vi "Neutral_ScanAgilentTrim_20170616.vi"(0 "Agilent E3631A Settings":T6={"VISA resource name"="GPIB0::5::INSTR", "Voltage Set (6V max)"=6.0, "Current Set (5A max)"=0.007, "Voltage Set (25V max)"=25.0, "Current Set (1A max)"=0.225, "Voltage Set (-25V max)"=25.0, "Current Set (1A max)"=0.225, "6V Switch"=FALSE, "+25V Switch"=FALSE, "-25V Switch"=FALSE, "Agilent E3631A Measurements"={"6V Actual Voltage Level (V)"=0.03231557, "6V Actual Current Level (A)"=0.01701259, "25V Actual Voltage Level (V)"=0.4256878, "25V Actual Current Level (A)"=0.2772881, "-25V Actual Current Level (A)"=0.0, "-25V Actual Voltage Level (V)"=0.0}, "Triggered Agilent Settings"={"Trigger \nDelay (s)"=3.0, "Enable +6V Channel"=TRUE, "+6V Current"=0.02, "Enable -25V Channel"=FALSE, "-25V Current"=0.0, "Enable +25V Channel"=TRUE, "+25V Current"=0.275}, "Auto Program Agilent"=FALSE, "Agilent Software Trigger"=FALSE} {"Triggered Agilent Settings"."Trigger \nDelay (s)" min=0.0 max=3600.0 step=1.0 format="%.2f"; "Agilent E3631A Measurements"."-25V Actual Current Level (A)" format="%.3g"; "Agilent E3631A Measurements"."-25V Actual Voltage Level (V)" format="%.3g"; "Agilent E3631A Measurements"."25V Actual Current Level (A)" format="%.3g"; "Agilent E3631A Measurements"."25V Actual Voltage Level (V)" format="%.3g"; "Agilent E3631A Measurements"."6V Actual Current Level (A)" format="%.3g"; "Agilent E3631A Measurements"."6V Actual Voltage Level (V)" format="%.3g"; "Current Set (1A max)" format="%.3g"; "Voltage Set (-25V max)" format="%.3g"; "Current Set (1A max)" format="%.3g"; "Voltage Set (25V max)" format="%.3g"; "Current Set (5A max)" format="%.3g"; "Voltage Set (6V max)" format="%.3g"}, 1 "Scan Parameters":T1={"Initial Values"=[81.5, 1.0, -0.1, 1.0], "Final Values"=[82.5, 3.0, 0.075, 5.0], "Step Sizes"=[0.015, 1.0, 0.025, 1.0], "Parameters to Change"=[enum."Synth Frequency", enum."Dummy Variable", enum."Red Mot 87 Initial Voltage", enum."Dummy Variable"], "Channels to Change"=[2, 0, 7, 0], "Number of Parameters to Scan"=2, "Parameter Nickname (no spaces)"=["", "ScanNo-", "Z-", "ScanNo-"], "Scan Base Name"="88Sr_3P1Spec_BFieldZero_X-0.02A_Y-0.277A_Z-0.6A_", "Raw_Data Folder"=path "\\\\mercury\\Neutral_Experiment/Raw_Data/2017.06.15", "ROI Parameters"={"Background Radius"=150.0, "Atom Radius"=120.0, "X Center"=365.0, "Y Center"=460.0}, "Drop Time (ms)"=17.0, "Phases To Change"=[1, 0, 2, 0], "Scan Pulseblaster Channel With Parameter"={"Change PB Time Toggle"=FALSE, "PB Channel"=10.0, "Parameter Number"=0.0}, "Preserve Waveform\nContinuity"=FALSE, "Generated Array Type"=enum."Default (old way)", "Master Batch Third Column"=0.277, "Master Batch Fourth Column"=0.0, "Master Batch Fifth Column"=0.0, "Current Param. Values"=[81.5, 1.0]} {"Current Param. Values" format="%^#.3e"; "Drop Time (ms)" min=1.0; "Number of Parameters to Scan" min=1}, 2 "Control Reference Cluster Input":T5, 3 "error in (no error)":errorcluster={"status"=FALSE, "code"=0, "source"="gettemp.vi: No error - function call successful"}) -> (10 "Error Out":errorcluster)   [LabVIEW 2016]
uses:
  Controls/Agilent E3631A/Settings_Control.ctl
  Controls/Agilent E3631A/Measurement_Indicator.ctl
  Controls/Agilent E3631A/Trigger_Settings.ctl
  Controls/ScanParameters/ScanParametersPanel.ctl
  Controls/ScanParameters/ParameterToChange.ctl
  Controls/ScanParameters/ROI_set.ctl
  Controls/ScanParameters/ScanPBandParam.ctl
panel:
  # "Select a PB Channel to set with a phase time for evaporation or whatever"
  # "Since the Agilent is slow to communicate the program will skip programming if the \"Auto Program Agilent\" switch is disabled.  If \"Auto Program\" is enabled the settings to the far left are used to program the Agilent.\n\nAdditionally, the Agilent has an internal software trigger that can a single channel between two current setpoints. The clock is not referenced to the Pulseblaster so be careful with timing when using the Triggered Agilent Settings. To enabled this mode use the \"Agilent Software Trigger\" swithc.\n\nUse the \"Program Agilent\" button to perform a one-time write (with settings on the far left) to avoid having the slow response of the supply during data scans.\n\nNOTE: When setting only current values the program will default to setting the maximum allowed voltage for a given channel."
  # "6V (2017.06.15)\n\nReported Current = \nSet Cur - 0.003A\n\nActual Current = \nSet Cur - 0.0015A"
  # "+25V (2017.06.15)\n\nReported Current = \nSet Cur + 0.002A\n\nActual Current = \nSet Cur + 0.002A"
  # "-25V (2017.06.15)\n\nReported Current = \nSet Cur\n\nActual Current = \nSet Cur"
  # "Beware of the offset in set, reported and actual current from Agilent channels. Below are corrections measured for each channel"
  # "--25V  Measurements"
  # "+25V  Measurements"
  # "6V  Measurements"
  # "-25V Output Settings"
  # "+25V Output Settings"
  # "6V Output Settings"
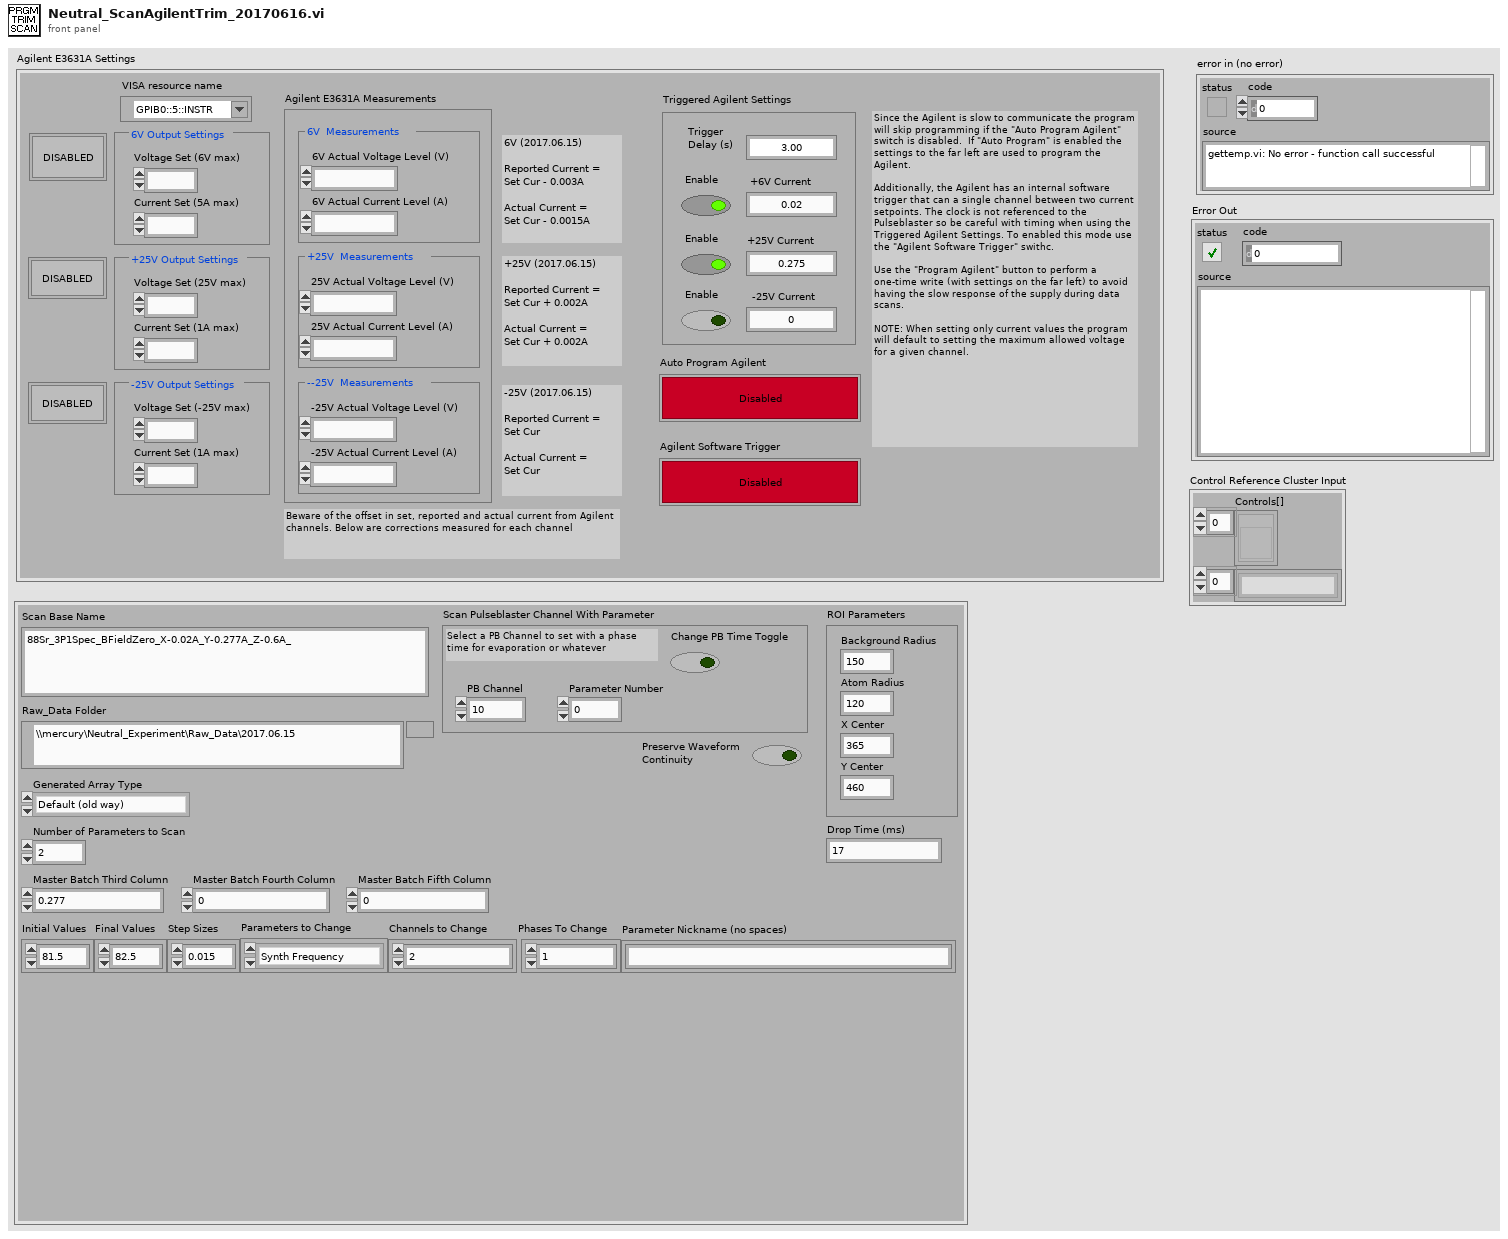
[diagram p1: front panel]
types:
  T1 = typedef "ScanParametersPanel.ctl" = cluster{"Initial Values":dbl[], "Final Values":dbl[], "Step Sizes":dbl[], "Parameters to Change":T2[], "Channels to Change":u32[], "Number of Parameters to Scan":i32, "Parameter Nickname (no spaces)":string[], "Scan Base Name":string, "Raw_Data Folder":path, "ROI Parameters":T3, "Drop Time (ms)":dbl, "Phases To Change":u32[], "Scan Pulseblaster Channel With Parameter":T4, "Preserve Waveform\nContinuity":bool, "Generated Array Type":enum16{"Custom Array From File", "Default (old way)"}, "Master Batch Third Column":dbl, "Master Batch Fourth Column":dbl, "Master Batch Fifth Column":dbl, "Current Param. Values":dbl[]}
  T2 = typedef "ParameterToChange.ctl" = enum16{"Dummy Variable", "Synth Amplitude", "Synth Frequency", "Synth Phase", "ODT Params Phase Time", "ODT Params Tau", "ODT Params Final Voltage", "ODT Params Initial Voltage", "ODT Params Eta", "Red Mot 88 Phase Time", "Red Mot 87 Phase Time", "Red Mot 88 Final Voltage", "Red Mot 88 Initial Voltage", "Red Mot 87 Final Voltage", "Red Mot 87 Initial Voltage", "PulseBlaster", "6713 Voltage", "Green Lattice Phase Time", "Green Lattice Initial Voltage", "Green Lattice Final Voltage", "Agilent Current Setpoint", "FPGA - Constant Op - Set", "FPGA - Bool Op - Output HI", "FPGA - Bool Op - Output LO", "FPGA - Custom Op"}
  T3 = typedef "ROI_set.ctl" = cluster{"Background Radius":dbl, "Atom Radius":dbl, "X Center":dbl, "Y Center":dbl}
  T4 = typedef "ScanPBandParam.ctl" = cluster{"Change PB Time Toggle":bool, "PB Channel":dbl, "Parameter Number":dbl}
  T5 = cluster{"Controls[]":refnum<vi>[], "Control Names":string[]}
  T6 = typedef "Settings_Control.ctl" = cluster{"VISA resource name":refnum<visa-resource-name>, "Voltage Set (6V max)":dbl, "Current Set (5A max)":dbl, "Voltage Set (25V max)":dbl, "Current Set (1A max)":dbl, "Voltage Set (-25V max)":dbl, "Current Set (1A max)":dbl, "6V Switch":bool, "+25V Switch":bool, "-25V Switch":bool, "Agilent E3631A Measurements":T7, "Triggered Agilent Settings":T8, "Auto Program Agilent":bool, "Agilent Software Trigger":bool}
  T7 = typedef "Measurement_Indicator.ctl" = cluster{"6V Actual Voltage Level (V)":dbl, "6V Actual Current Level (A)":dbl, "25V Actual Voltage Level (V)":dbl, "25V Actual Current Level (A)":dbl, "-25V Actual Current Level (A)":dbl, "-25V Actual Voltage Level (V)":dbl}
  T8 = typedef "Trigger_Settings.ctl" = cluster{"Trigger \nDelay (s)":dbl, "Enable +6V Channel":bool, "+6V Current":dbl, "Enable -25V Channel":bool, "-25V Current":dbl, "Enable +25V Channel":bool, "+25V Current":dbl}
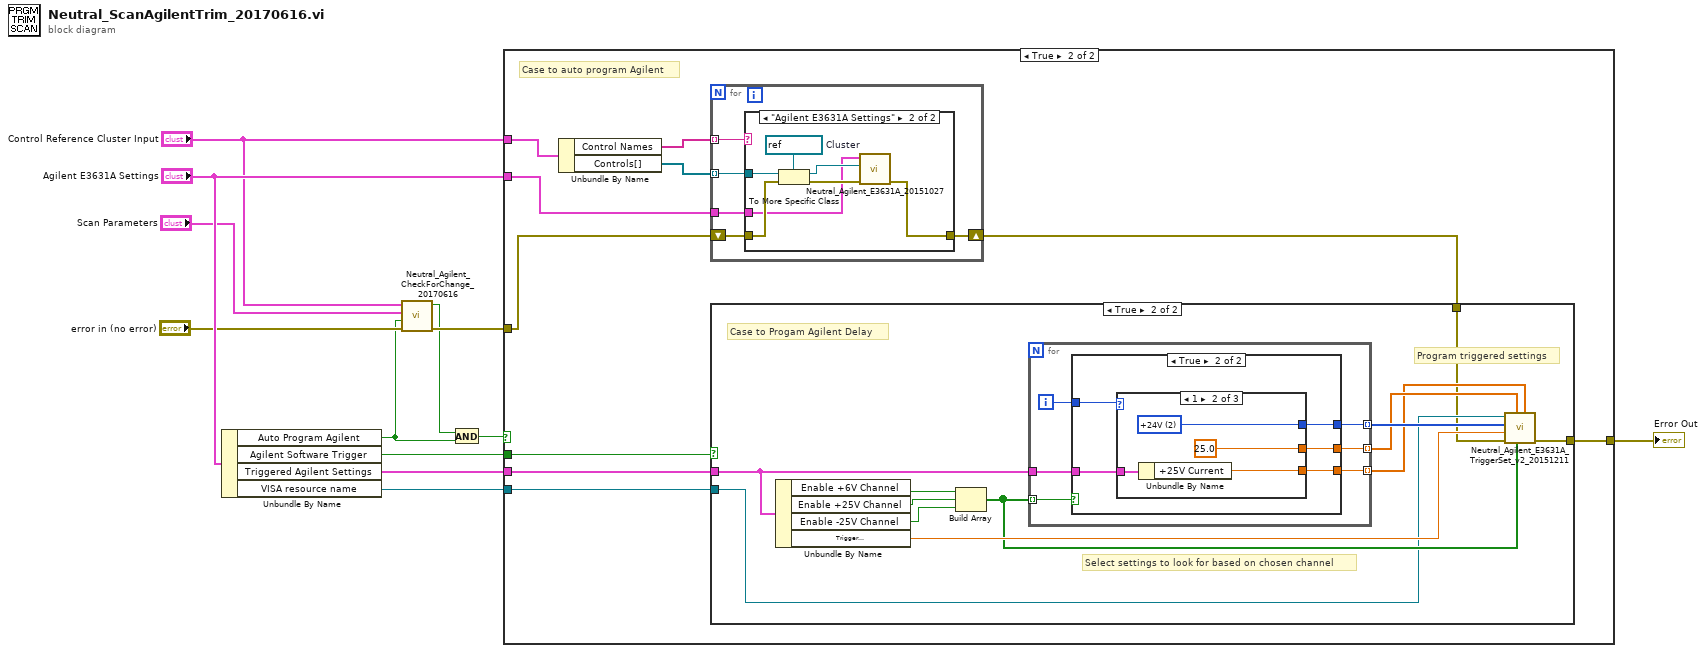
[diagram p0: block diagram]
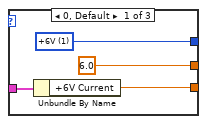
[diagram p6: hidden frame]
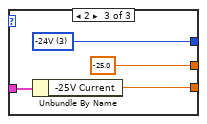
[diagram p7: hidden frame]
diagram:
  n1 = Unbundle By Name("Agilent E3631A Settings") -> ("Auto Program Agilent"=w2:bool, "Agilent Software Trigger"=w8:bool, "Triggered Agilent Settings"=w11:T8, "VISA resource name"=w9:refnum<visa-resource-name>)
  n2 = call "Neutral_Agilent_CheckForChange_20170616.vi"("Control Reference Cluster Input"="Control Reference Cluster Input", "Scan Parameters"="Scan Parameters", "Auto Program Agilent"=w2, "error in (no error)"="error in (no error)") -> ("Changed Current?"=w1:bool, "Error Out"=w6:errorcluster)  [unwired: 5 in]
  n3 = And(x=w1, y=w2) -> (x .and. y?=w3:bool)
  n4 = case shown="True" w3 {
    tunnel: "Agilent E3631A Settings" -> [_ w14]
    tunnel: w11 -> [_ w23]
    tunnel: w6 -> [w13 w15]
    tunnel: [w13 w22] -> w12
    tunnel: w9 -> [_ w21]
    tunnel: w8 -> [_ w20]
    tunnel: "Control Reference Cluster Input" -> [_ w16]
    frame False {
    }
    frame True {
      # "Case to auto program Agilent"
      n5 = Unbundle By Name(w16) -> ("Control Names"=w18:string[], "Controls[]"=w19:refnum<vi>[])
      n6 = for {
        tunnel: w18 -> [w28] mode=indexing
        shift-right: [w25] -> w17
        shift-left: w15 -> [w26]
        tunnel: w19 -> [w27] mode=indexing
        tunnel: w14 -> [w24]
        n7 = case shown="\"Agilent E3631A Settings\"" w28 {
          tunnel: w27 -> [_ w35]
          tunnel: w26 -> [w29 w32]
          tunnel: [w29 w36] -> w25
          tunnel: w24 -> [_ w30]
          frame "False", Default {
          }
          frame "Agilent E3631A Settings" {
            w34 = refnum<vi> refnum  # Cluster
            n8 = To More Specific Class(target class=w34, reference=w35, error in=w32) -> (specific class reference=w33:refnum<vi>, error out=w31:errorcluster)
            n9 = call "Neutral_Agilent_E3631A_20151027.vi"("error in (no error)"=w31, "Agilent E3631A RefNum"=w33, "Agilent E3631A Settings"=w30) -> ("error out"=w36:errorcluster)  [unwired: 8 in]
          }
        }
      }
      n10 = case shown="True" w20 {
        tunnel: w23 -> [_ w46]
        tunnel: [w37 w40] -> w22
        tunnel: w21 -> [_ w39]
        tunnel: w17 -> [w37 w38]
        frame False {
        }
        frame True {
          # "Case to Progam Agilent Delay"
          # "Program triggered settings"
          # "Select settings to look for based on chosen channel"
          n11 = Unbundle By Name(w46) -> ("Enable +6V Channel"=w49:bool, "Enable +25V Channel"=w48:bool, "Enable -25V Channel"=w47:bool, "Trigger \nDelay (s)"=w44:dbl)
          n12 = Build Array(w49, w48, w47) -> (w41:bool[])
          n13 = for {
            tunnel: [w54] -> w42 mode=indexing
            tunnel: [w53] -> w45 mode=indexing
            tunnel: w41 -> [w52] mode=indexing
            tunnel: w46 -> [w51]
            tunnel: [w50] -> w43 mode=indexing
            i -> [w55]
            n14 = case shown="True" w52 {
              tunnel: w55 -> [_ w60]
              tunnel: [_ w59] -> w54
              tunnel: [_ w58] -> w53
              tunnel: w51 -> [_ w57]
              tunnel: [_ w56] -> w50
              frame False {
              }
              frame True {
                n15 = case shown="1" w60 {
                  tunnel: [w64 w68 w72] -> w59
                  tunnel: [w63 w67 w71] -> w58
                  tunnel: w57 -> [w62 w66 w70]
                  tunnel: [6.0 ("Voltage Set (-25V max)") 25.0 ("Voltage Set (25V max)") -25.0 ("Voltage Set (25V max)")] -> w56
                  frame 0, Default {
                    w63 = 1 items=["+6V"=1, "+24V"=2, "-24V"=3] ("Channel")
                    n16 = Unbundle By Name(w62) -> ("+6V Current"=w64:dbl)
                  }
                  frame 1 {
                    w67 = 2 items=["+6V"=1, "+24V"=2, "-24V"=3] ("Channel")
                    n17 = Unbundle By Name(w66) -> ("+25V Current"=w68:dbl)
                  }
                  frame 2 {
                    w71 = 3 items=["+6V"=1, "+24V"=2, "-24V"=3] ("Channel")
                    n18 = Unbundle By Name(w70) -> ("-25V Current"=w72:dbl)
                  }
                }
              }
            }
          }
          n19 = call "Neutral_Agilent_E3631A_TriggerSet_v2_20151211.vi"("Triggeed Current Limit"=w42, "Program Trigger?"=w41, "Triggerd Voltage Level"=w43, "error in (no error)"=w38, "Trigger Delay (s)"=w44, "Channel"=w45, "VISA resource name"=w39) -> ("error out"=w40:errorcluster)  [unwired: 4 in]
        }
      }
    }
  }
  "Error Out" <- w12
